vi "lv_mysql_conn_init.vi"(6 "timeout ms (5000)":i32=5000, 8 "error in (no error)":errorcluster, 9 "Authentication":T1, 10 "Port":u16=3306, 11 "IP Address":string) -> (0 "error out":errorcluster, 3 "connection ID out":refnum<k5>)   [LabVIEW 2010]
uses:
  typedefs/mysql_authentication.ctl
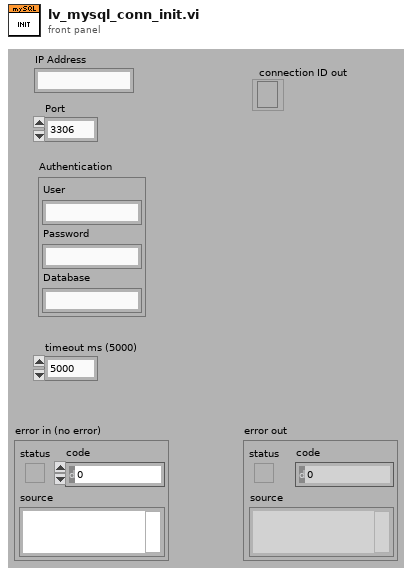
[diagram p1: front panel]
types:
  T1 = typedef "mysql_authentication.ctl" = cluster{"User":string, "Password":string, "Database":string}
  T2 = typedef "Server_Init_Data.ctl" = cluster{"Protocol Version":u8, "Server Version":string, "Thread ID":u32, "Scramble Buffer":u8[], "Server Capabilities":u16, "Server Languague":u8, "Server Status":u16}
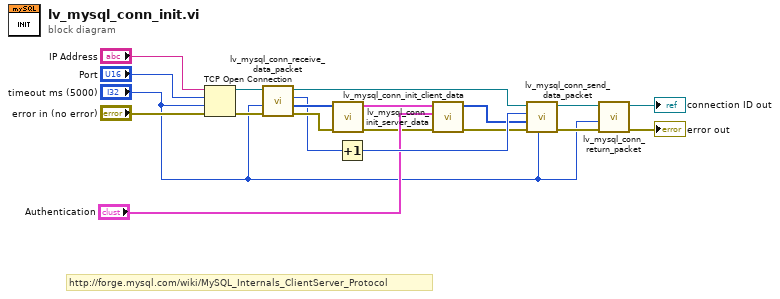
[diagram p0: block diagram]
diagram:
  # "http://forge.mysql.com/wiki/MySQL_Internals_ClientServer_Protocol"
  n1 = TCP Open Connection(address="IP Address", remote port or service name="Port", timeout ms (60000)="timeout ms (5000)", error in (no error)="error in (no error)") -> (connection ID=w15:refnum<k5>, error out=w16:errorcluster)  [unwired: 1 in]
  n2 = call "lv_mysql_conn_receive_data_packet.vi"("error in"=w16, "timeout ms (5000)"="timeout ms (5000)", "connection ID"=w15) -> ("error out"=w18:errorcluster, "TCP/IP Data"=w14:u8[], "Packet #"=w11:u8, "connection ID out"=w12:refnum<k5>)  [unwired: 5 in]
  n3 = call "lv_mysql_conn_init_server_data.vi"("error in (no error)"=w18, "TCPIP Data"=w14) -> ("error out"=w8:errorcluster, "Server Init Data"=w9:T2)  [unwired: 8 in]
  n4 = Increment(x=w11) -> (x+1=w13:u8)
  n5 = call "lv_mysql_conn_init_client_data.vi"("error in (no error)"=w8, "Authentication"="Authentication", "Server Init Data"=w9) -> ("error out"=w7:errorcluster, "TCPIP Data"=w6:u8[])  [unwired: 7 in]
  n6 = call "lv_mysql_conn_send_data_packet.vi"("timeout ms (5000)"="timeout ms (5000)", "error in"=w7, "TCP/IP Data"=w6, "Packet #"=w13, "connection ID"=w12) -> ("error out"=w4:errorcluster, "connection ID out"=w2:refnum<k5>)  [unwired: 5 in]
  n7 = call "lv_mysql_conn_return_packet.vi"("error in (no error)"=w4, "timeout ms (5000)"="timeout ms (5000)", "connection ID"=w2) -> ("error out"=→"error out":errorcluster, "connection ID out"=→"connection ID out":refnum<k5>)  [unwired: 5 in, 2 out]
